vi "getData.vi"(8 "error in (no error)":errorcluster, 11 "DeviceData in":refnum<class "DeviceData.lvclass">) -> (0 "error out":errorcluster, 1 "dataArray":dbl[][](array[numeric]), 2 "data out":T1(array[cluster]) {"time" format="%_8g"}, 3 "DeviceData out":refnum<class "DeviceData.lvclass">, 4 "times":dbl[](array[numeric]), 5 "soundStreamPath":path)   [LabVIEW 2011, in "DataMappers.lvlib" / "DeviceData.lvclass"]
uses:
  DeviceData.lvclass
  DatabaseHelpers/Database Objects/Channel/Channel.lvclass
  DeviceData.lvclass/DeviceData.ctl
  SoundDeviceData/SoundDeviceData.lvclass
  DatabaseHelpers/Database Objects/device/device.lvclass
  Scripting/ScriptingEvent/ScriptEventList/ScriptEventList.lvclass
panel:
  out "Array 3":dbl[][](array[numeric])
  out "Array 2":string[][](array[string])
  out "Array":dbl[][](array[numeric])
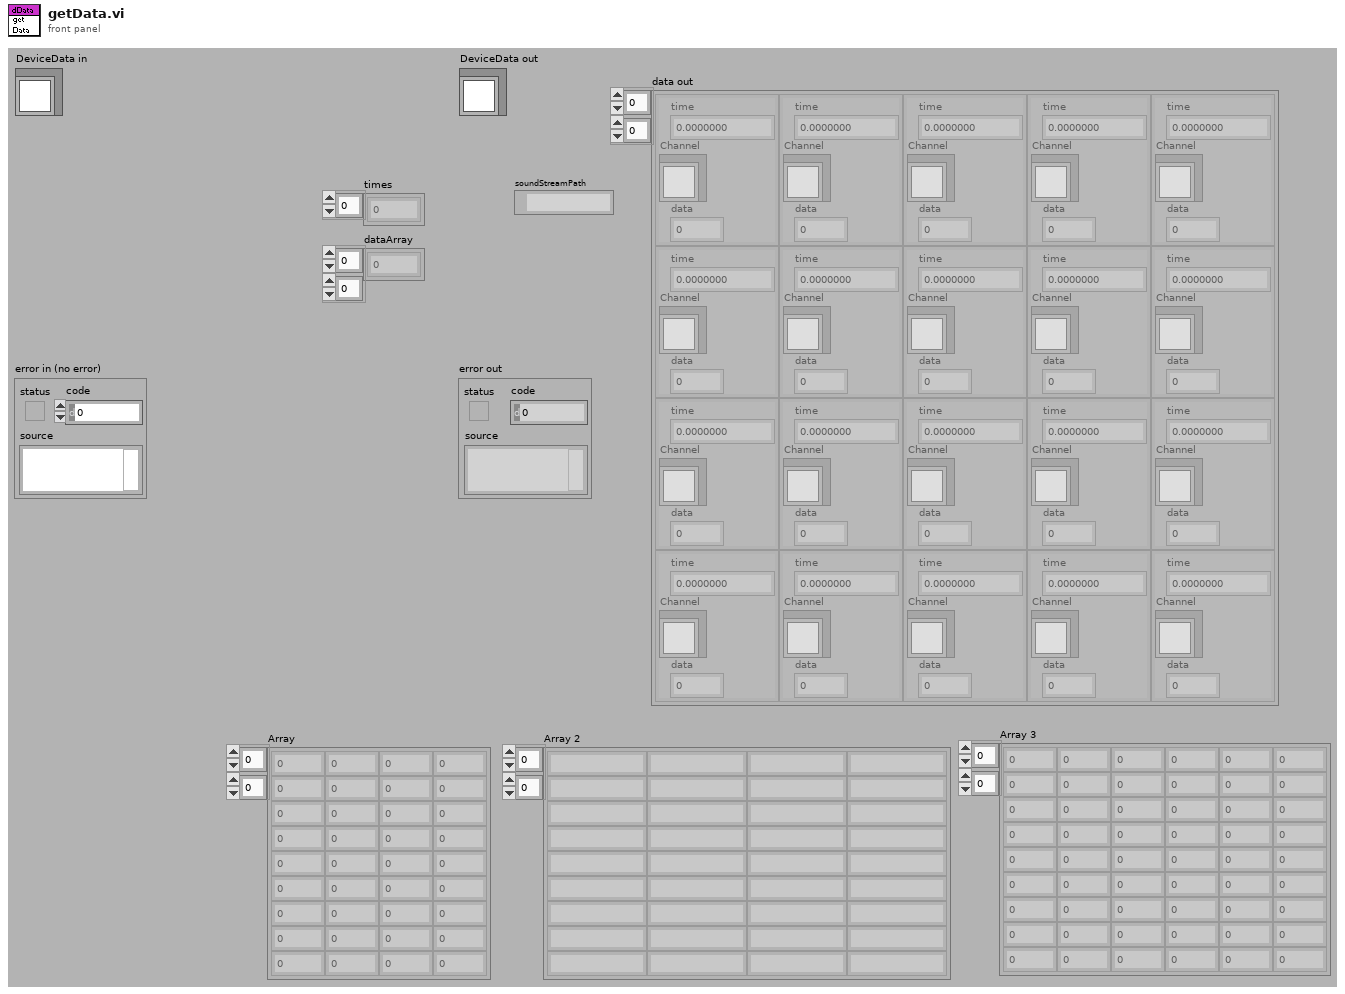
[diagram p1: front panel]
types:
  T1 = cluster{"time":dbl, "Channel":refnum<class "Channel.lvclass">, "data":dbl}[][]
  T2 = cluster{"time":dbl, "Channel":refnum<class "Channel.lvclass">, "value":dbl}[][]
  T3 = cluster{"Channel":refnum<class "Channel.lvclass">, "time":dbl[], "Amplitude":dbl[], "frequency":dbl[], "phase":dbl[]}[]
  T4 = enum16{"eventData", "singleToneData", "fileData"}
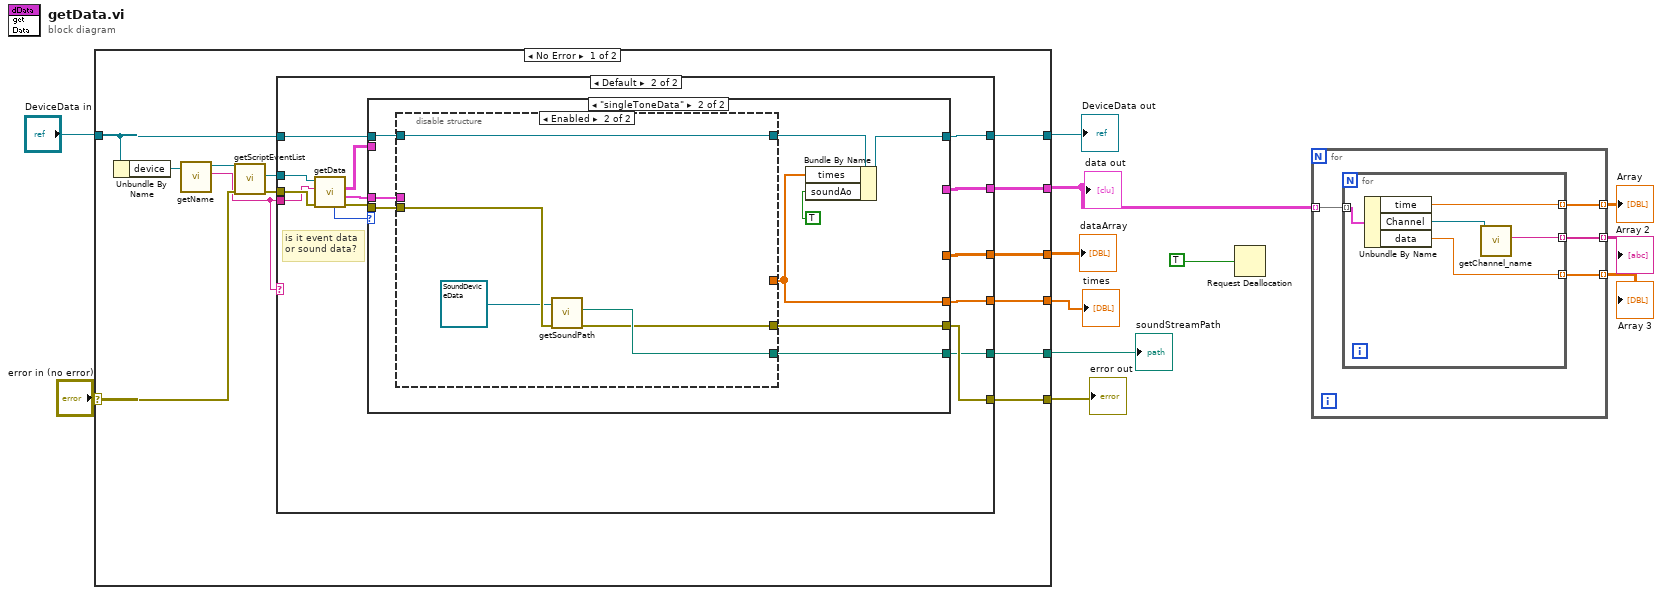
[diagram p0: block diagram]
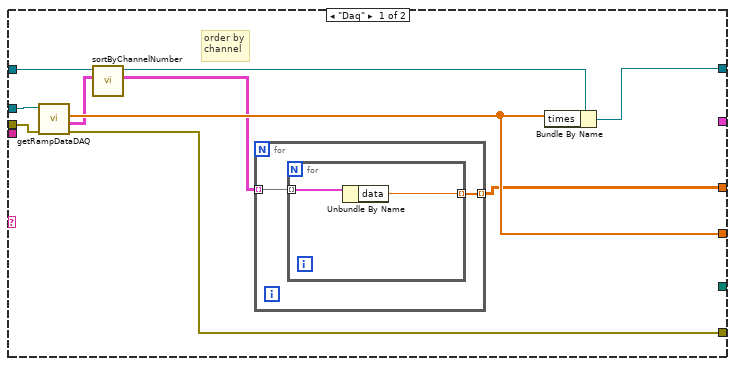
[diagram p2: hidden frame]
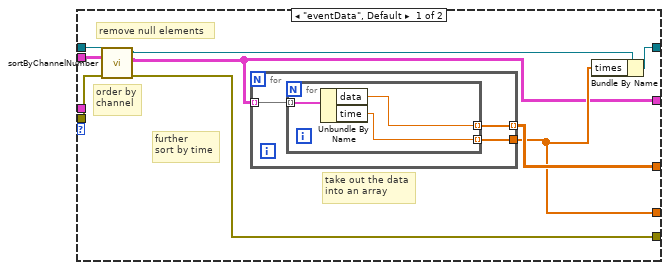
[diagram p3: hidden frame]
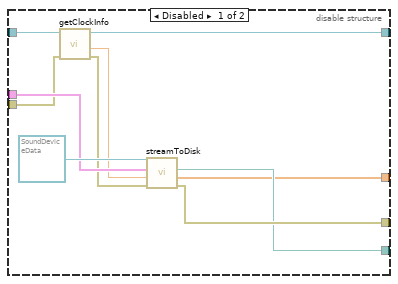
[diagram p4: hidden frame]
diagram:
  n1 = case shown="No Error" "error in (no error)" {
    selector: "error in (no error)" -> [w25 w94]
    tunnel: [w20 w94] -> w11
    tunnel: [w18 w93] -> w9
    tunnel: "DeviceData in" -> [w19 w93]
    tunnel: [w21 _] -> w4
    tunnel: [w22 _] -> w8
    tunnel: [w17 _] -> w7
    tunnel: [w16 _] -> w5
    frame No Error {
      n2 = Unbundle By Name(w19) -> ("device"=w14:refnum<class "device.lvclass">)
      n3 = call "getName.vi"("device.lvclass in"=w14) -> ("name"=w13:string, "device.lvclass out"=w15:refnum<class "device.lvclass">)  [unwired: 8 in, 1 out]
      n4 = call "getScriptEventList.vi"("error in (no error)"=w25, "device.lvclass in"=w15) -> ("error out"=w23:errorcluster, "ScriptEventList"=w24:refnum<class "ScriptEventList.lvclass">)  [unwired: 7 in, 1 out]
      n5 = case shown="Default" w13 {
        tunnel: w24 -> [w35 w53]
        tunnel: w23 -> [w34 w52]
        tunnel: [w26 w51] -> w22
        tunnel: [_ w50] -> w21
        tunnel: [w33 w49] -> w20
        tunnel: w19 -> [w30 w48]
        tunnel: [w31 w45] -> w18
        tunnel: [w32 w44] -> w17
        tunnel: [_ w41] -> w16
        tunnel: w13 -> [_ w40]
        frame "Daq" {
          # "order by\nchannel"
          n6 = call "getRampDataDAQ.vi"("error in (no error)"=w34, "ScriptEventList in"=w35) -> ("error out"=w33:errorcluster, "data out"=w29:T2, "times out"=w32:dbl[])  [unwired: 6 in, 1 out]
          n7 = call "sortByChannelNumber.vi"("data in"=w29, "DeviceData in"=w30) -> ("data out"=w27:T1, "DeviceData out"=w28:refnum<class "DeviceData.lvclass">)  [unwired: 7 in, 1 out]
          n8 = for {
            tunnel: w27 -> [w37] mode=indexing
            tunnel: [w36] -> w26 mode=indexing
            n9 = for {
              tunnel: w37 -> [w39] mode=indexing
              tunnel: [w38] -> w36 mode=indexing
              n10 = Unbundle By Name(w39) -> ("data"=w38:dbl)
            }
          }
          n11 = Bundle By Name(cluster=w28, "times"=w32) -> (w31:refnum<class "DeviceData.lvclass">)
        }
        frame Default {
          # "is it event data\nor sound data?"
          n12 = call "getData.vi"("error in (no error)"=w52, "device_name"=w40, "ScriptEventList in"=w53) -> ("error out"=w46:errorcluster, "singleToneData"=w42:T3, "data out"=w47:T1, "dataType"=w43:T4)  [unwired: 4 in, 1 out]
          n13 = case shown="\"singleToneData\"" w43 {
            tunnel: [w62 _] -> w51
            tunnel: [w54 _] -> w50
            tunnel: [w57 w74] -> w49
            tunnel: w48 -> [w58 w71]
            tunnel: w47 -> [w60 _]
            tunnel: w46 -> [w59 w69]
            tunnel: [w56 w77] -> w45
            tunnel: [w61 w72] -> w44
            tunnel: w42 -> [_ w75]
            tunnel: [_ w73] -> w41
            frame "eventData", Default {
              # "take out the data\ninto an array"
              # "further\nsort by time"
              # "order by\nchannel"
              # "remove null elements"
              n14 = call "sortByChannelNumber.vi"("error in (no error)"=w59, "data in"=w60, "DeviceData in"=w58) -> ("error out"=w57:errorcluster, "data out"=w54:T1, "DeviceData out"=w55:refnum<class "DeviceData.lvclass">)  [unwired: 6 in]
              n15 = for {
                tunnel: w54 -> [w65] mode=indexing
                tunnel: [w64] -> w62 mode=indexing
                tunnel: [w63] -> w61
                n16 = for {
                  tunnel: w65 -> [w68] mode=indexing
                  tunnel: [w67] -> w64 mode=indexing
                  tunnel: [w66] -> w63 mode=indexing
                  n17 = Unbundle By Name(w68) -> ("data"=w67:dbl, "time"=w66:dbl)
                }
              }
              n18 = Bundle By Name(cluster=w55, "times"=w61) -> (w56:refnum<class "DeviceData.lvclass">)
            }
            frame "singleToneData" {
              n19 = disable-structure shown="Enabled" {
                disable-tunnel: w75 -> [w86 _]
                disable-tunnel: [w85 w89] -> w74
                disable-tunnel: [w84 w91] -> w73
                disable-tunnel: [w83 _] -> w72
                disable-tunnel: w71 -> [w82 w92]
                disable-tunnel: [w80 w92] -> w70
                disable-tunnel: w69 -> [w79 w90]
                frame Disabled {
                  n20 = call "getClockInfo.vi"("error in (no error)"=w79, "DeviceData in"=w82) -> ("error out"=w78:errorcluster, "masterClockRate"=w81:dbl, "DeviceData out"=w80:refnum<class "DeviceData.lvclass">)  [unwired: 5 in, 2 out]
                  n21 = call "streamToDisk.vi"("error in (no error)"=w78, "sampleRate"=w81, "singleToneData"=w86, "SoundDeviceData in"=refnum<class "SoundDeviceData.lvclass"> refnum ("DataMappers.lvlib:SoundDeviceData.lvclass")) -> ("error out"=w85:errorcluster, "times"=w83:dbl[], "Path"=w84:path)  [unwired: 4 in, 1 out]
                }
                frame Enabled {
                  n22 = call "getSoundPath.vi"("error in (no error)"=w90, "SoundDeviceData in"=refnum<class "SoundDeviceData.lvclass"> refnum ("DataMappers.lvlib:SoundDeviceData.lvclass")) -> ("error out"=w89:errorcluster, "Path"=w91:path)  [unwired: 7 in, 1 out]
                }
              }
              n23 = Bundle By Name(cluster=w70, "times"=w72, "soundAo"=TRUE) -> (w77:refnum<class "DeviceData.lvclass">)
            }
          }
        }
      }
    }
    frame Error {
    }
  }
  "error out" <- w11
  "DeviceData out" <- w9
  "data out" <- w4
  "dataArray" <- w8
  "times" <- w7
  "soundStreamPath" <- w5
  n24 = Request Deallocation(TRUE) -> ()
  n25 = for {
    tunnel: w4 -> [w98] mode=indexing
    tunnel: [w97] -> w3 mode=indexing
    tunnel: [w96] -> w2 mode=indexing
    tunnel: [w95] -> w1 mode=indexing
    n26 = for {
      tunnel: w98 -> [w103] mode=indexing
      tunnel: [w102] -> w97 mode=indexing
      tunnel: [w100] -> w96 mode=indexing
      tunnel: [w99] -> w95 mode=indexing
      n27 = Unbundle By Name(w103) -> ("time"=w102:dbl, "Channel"=w101:refnum<class "Channel.lvclass">, "data"=w99:dbl)
      n28 = call "getChannel_name.vi"("Channel.lvclass in"=w101) -> ("channel_name"=w100:string)  [unwired: 8 in, 2 out]
    }
  }
  "Array" <- w3
  "Array 2" <- w2
  "Array 3" <- w1
